vi "Threshold.vi"(0 "image in":refnum<class "MSC Image.lvclass">, 1 "ThresholdLow":dbl, 2 "ThresholdHigh":dbl=100.0, 5 "error in (no error)":errorcluster) -> (14 "image out":refnum<class "MSC Image.lvclass">, 19 "error out":errorcluster)   [LabVIEW 2014, in "MSC Image.lvclass"]
doc: "Applies a threshold to the image. \n\nLow < High: Pixels between the borders are extracted\nLow > High: Pixels excluded by the borders are extracted"
uses:
  MSC Image.lvclass
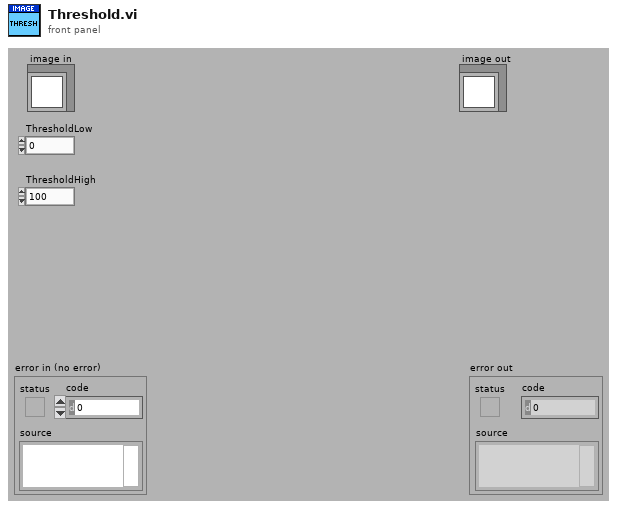
[diagram p1: front panel]
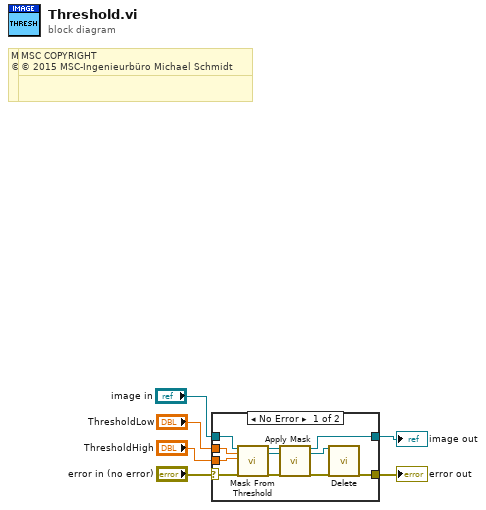
[diagram p0: block diagram]
diagram:
  # "MSC COPYRIGHT\n© 2016 MSC-Ingenieurbüro Michael Schmidt"
  # "MSC COPYRIGHT\n© 2016 MSC-Ingenieurbüro Michael Schmidt"
  # "MSC COPYRIGHT\n© 2015 MSC-Ingenieurbüro Michael Schmidt"
  # "MSC COPYRIGHT\n© 2015 MSC-Ingenieurbüro Michael Schmidt"
  n1 = case shown="No Error" "error in (no error)" {
    selector: "error in (no error)" -> [w7 w19]
    tunnel: [w13 w19] -> w5
    tunnel: [w17 w18] -> w3
    tunnel: "image in" -> [w10 w18]
    tunnel: "ThresholdLow" -> [w12 _]
    tunnel: "ThresholdHigh" -> [w11 _]
    frame No Error {
      n2 = call-dynamic "Mask From Threshold.vi"("image in"=w10, "Threshold Low"=w12, "Threshold High"=w11, "error in (no error)"=w7) -> ("image out"=w9:refnum<class "MSC Image.lvclass">, "mask image out"=w8:refnum<class "MSC Image.lvclass">, "error out"=w14:errorcluster)  [unwired: 13 in]
      n3 = call-dynamic "Apply Mask.vi"("image in"=w9, "mask image in"=w8, "error in (no error)"=w14) -> ("image out"=w17:refnum<class "MSC Image.lvclass">, "mask image out"=w16:refnum<class "MSC Image.lvclass">, "error out"=w15:errorcluster)  [unwired: 14 in]
      n4 = call-dynamic "Delete.vi"("image in"=w16, "error in (no error)"=w15) -> ("error out"=w13:errorcluster)  [unwired: 17 in]
    }
    frame Error {
    }
  }
  "error out" <- w5
  "image out" <- w3
